vi "Read Write License File.vi"(0 "License File Data":T1, 1 "License File Name":string="License.lic", 5 "License File Path":path, 11 "Error in (no error)":errorcluster, 13 "Operation":enum16{"Write", "Read"}(ring)=enum."Read") -> (4 "License File Data Out":T1, 6 "License File Path":path, 15 "Error out":errorcluster)   [LabVIEW 2022 SP3]
uses:
  Controls/License File Data.ctl
  Controls/License Types.ctl
  <vilib>/Utility/sysdir.llb/System Directory Type.ctl
panel:
  out "ROT'd string":string
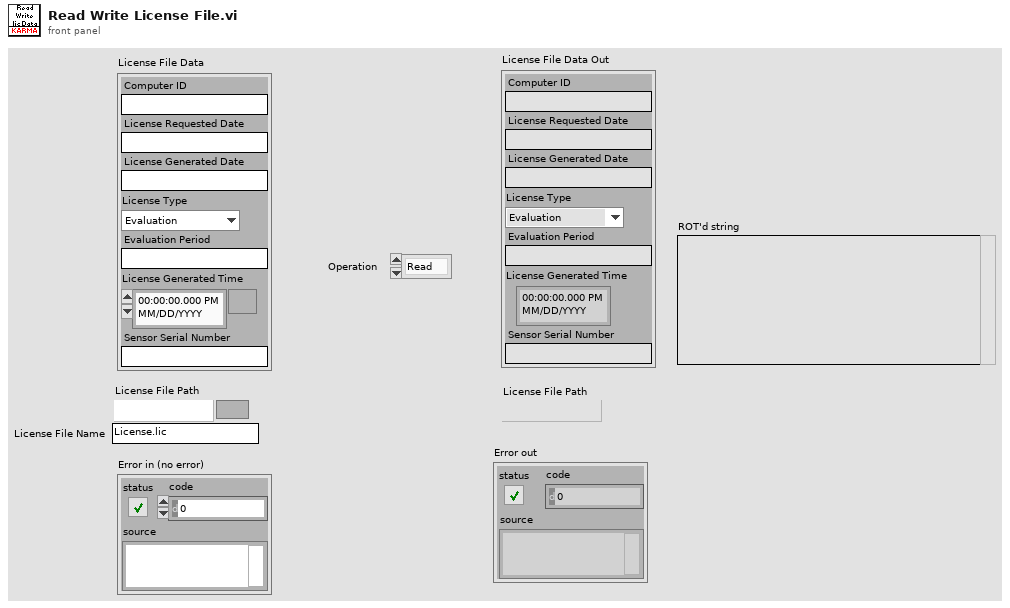
[diagram p1: front panel]
types:
  T1 = typedef "License File Data.ctl" = cluster{"Computer ID":string, "License Requested Date":string, "License Generated Date":string, "License Type":T2, "Evaluation Period":string, "License Generated Time":timestamp, "Sensor Serial Number":string}
  T2 = typedef "License Types.ctl" = enum16{"Evaluation", "Professional"}
  T3 = enum16{"open", "replace", "create", "open or create", "replace or create", "replace or create with confirmation"}
  T4 = typedef "System Directory Type.ctl" = i32
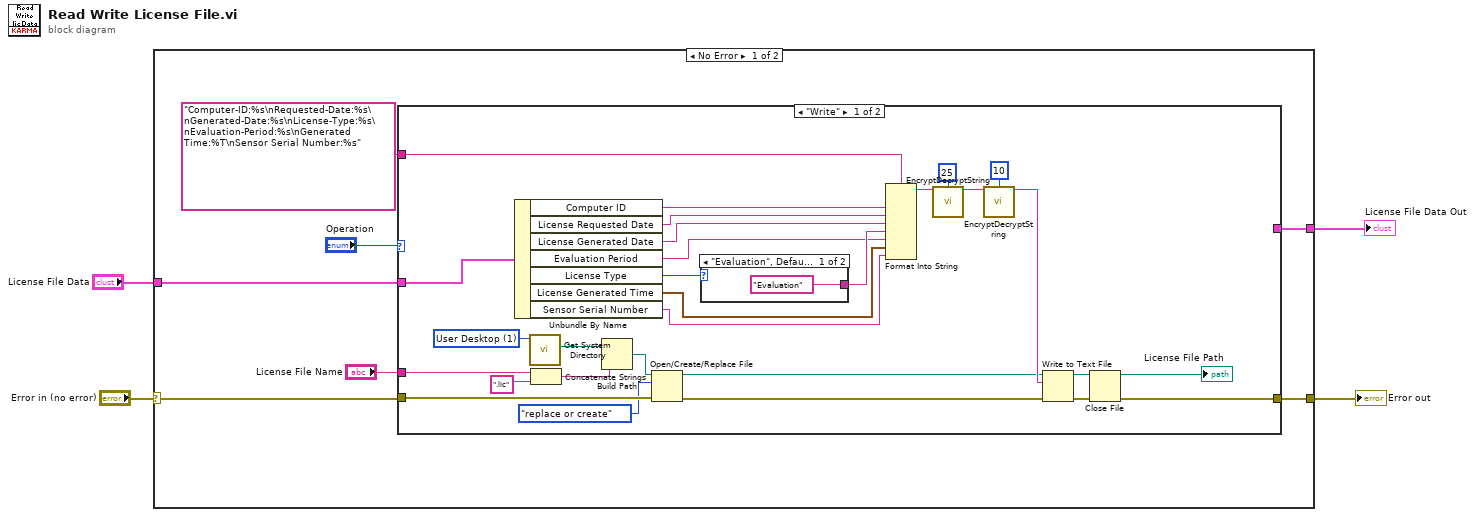
[diagram p0: block diagram]
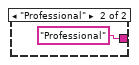
[diagram p2: hidden frame]
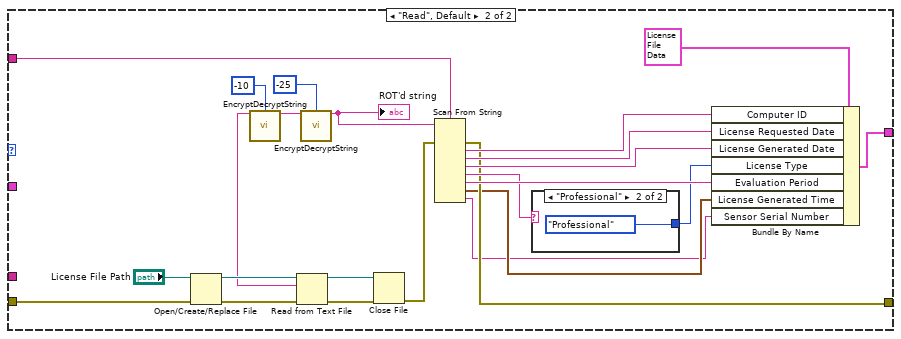
[diagram p3: hidden frame]
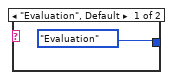
[diagram p4: hidden frame]
diagram:
  n1 = case shown="No Error" "Error in (no error)" {
    selector: "Error in (no error)" -> [w8 w69]
    tunnel: [w9 w69] -> w4
    tunnel: "License File Data" -> [w11 _]
    tunnel: [w5 _] -> w1
    frame No Error {
      n2 = case shown="\"Write\"" "Operation" {
        tunnel: w11 -> [w40 _]
        tunnel: [w23 w45] -> w9
        tunnel: w8 -> [w29 w62]
        tunnel: "Computer-ID:%s\nRequested-Date:%s\nGenerated-Date:%s\nLicense-Type:%s\nEvaluation-Period:%s\nGenerated Time:%T\nSensor Serial Number:%s" ("format string") -> [w21 w61]
        tunnel: "License File Name" -> [w19 _]
        tunnel: [_ w47] -> w5
        frame "Write" {
          w27 = T4 1 items=["User Home"=0, "User Desktop"=1, "User Documents"=2, "User Application Data"=3, "User Preferences"=4, "User Temporary"=5, "Public Documents"=6, "Public Application Data"=7, "Public Preferences"=8, "Public Cache"=13, "System Core Libraries"=9, "System Installed Libraries"=10, "Application Files"=11, "Boot Volume Root"=12] ("system directory type")
          n3 = Unbundle By Name(w40) -> ("Computer ID"=w39:string, "License Requested Date"=w38:string, "License Generated Date"=w37:string, "Evaluation Period"=w16:string, "License Type"=w17:T2, "License Generated Time"=w13:timestamp, "Sensor Serial Number"=w12:string)
          n4 = call <vilib>:"Get System Directory.vi"("system directory type"=w27) -> ("system directory"=w30:path)  [unwired: 10 in]
          n5 = Concatenate Strings(w19, ".lic" ("string")) -> (w15:string)
          n6 = Build Path(base path=w30, name or relative path=w15) -> (appended path=w31:path)
          n7 = Open/Create/Replace File(file path (use dialog)=w31, error in=w29, operation (0:open)=T3."replace or create") -> (refnum out=w25:refnum<file>, error out=w26:errorcluster)  [unwired: 3 in, 1 out]
          n8 = case shown="\"Evaluation\", Default" w17 {
            tunnel: ["Evaluation" "Professional"] -> w18
            frame "Evaluation", Default {
            }
            frame "Professional" {
            }
          }
          n9 = Format Into String(format string=w21, w39, w38, w37, w18, w16, w13, w12) -> (resulting string=w36:string)  [unwired: 2 in, 1 out]
          n10 = call "EncryptDecryptString.vi"("Original"=w36, "ROT by..."=25) -> ("ROT'd string"=w34:string)  [unwired: 13 in]
          n11 = call "EncryptDecryptString.vi"("Original"=w34, "ROT by..."=10) -> ("ROT'd string"=w32:string)  [unwired: 13 in]
          n12 = Write to Text File(file (use dialog)=w25, text=w32, error in=w26) -> (refnum out=w22:refnum<file>, error out=w24:errorcluster)  [unwired: 1 in, 1 out]
          n13 = Close File(refnum=w22, error in=w24) -> (path=→"License File Path":path, error out=w23:errorcluster)
        }
        frame "Read", Default {
          n14 = Open/Create/Replace File(file path (use dialog)="License File Path", error in=w62) -> (refnum out=w64:refnum<file>, error out=w66:errorcluster)  [unwired: 4 in, 1 out]
          n15 = Read from Text File(file (use dialog)=w64, error in=w66) -> (refnum out=w51:refnum<file>, text=w57:string, error out=w65:errorcluster)  [unwired: 2 in, 1 out]
          n16 = call "EncryptDecryptString.vi"("Original"=w57, "ROT by..."=-10) -> ("ROT'd string"=w58:string)  [unwired: 13 in]
          n17 = call "EncryptDecryptString.vi"("Original"=w58, "ROT by..."=-25) -> ("ROT'd string"=w56:string)  [unwired: 13 in]
          "ROT'd string" <- w56
          n18 = Close File(refnum=w51, error in=w65) -> (error out=w46:errorcluster)  [unwired: 1 out]
          n19 = Scan From String(format string=w61, input string=w56, error in=w46) -> (error out=w45:errorcluster, output 1=w55:string, output 2=w54:string, output 3=w53:string, output 4=w48:string, output 5=w52:string, output 6=w44:timestamp, output 7=w43:string)  [unwired: 8 in, 2 out]
          n20 = case shown="\"Professional\"" w48 {
            tunnel: [License_Types."Evaluation" ("License Type") License_Types."Professional" ("License Type")] -> w49
            frame "Evaluation", Default {
            }
            frame "Professional" {
            }
          }
          n21 = Bundle By Name(cluster=T1 {"Computer ID"="", "License Requested Date"="", "License Generated Date"="", "License Type"=enum."Evaluation", "Evaluation Period"="", "License Generated Time"=timestamp(0 s since 1904-01-01), "Sensor Serial Number"=""} ("License File Data"), "Computer ID"=w55, "License Requested Date"=w54, "License Generated Date"=w53, "License Type"=w49, "Evaluation Period"=w52, "License Generated Time"=w44, "Sensor Serial Number"=w43) -> (w47:T1)
        }
      }
    }
    frame Error {
    }
  }
  "Error out" <- w4
  "License File Data Out" <- w1
